vi "Quadratic Roots.vi"() -> ()   [LabVIEW 2021]
panel:
  out "Root 2":dbl
  out "Root 1":dbl
  in  "C":dbl
  in  "B":dbl
  in  "A":dbl
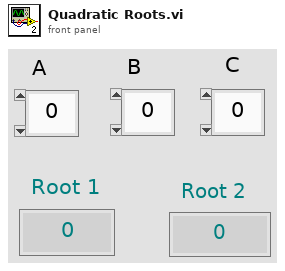
[diagram p1: front panel]
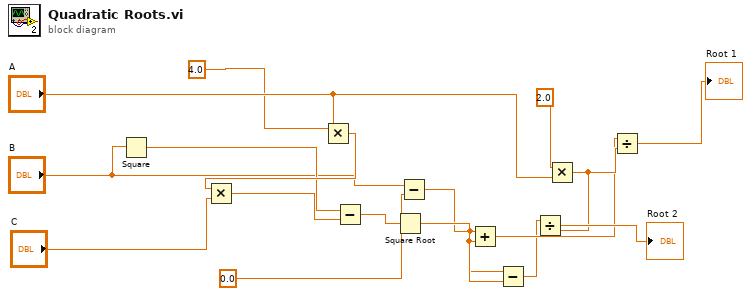
[diagram p0: block diagram]
diagram:
  n1 = Square(x="B") -> (x^2=w15:dbl)
  n2 = Multiply(x=4.0, y="A") -> (x*y=w17:dbl)
  n3 = Multiply(x=w17, y="C") -> (x*y=w14:dbl)
  n4 = Subtract(x=w15, y=w14) -> (x-y=w13:dbl)
  n5 = Square Root(x=w13) -> (sqrt(x)=w7:dbl)
  n6 = Subtract(x="B", y=0.0) -> (x-y=w6:dbl)
  n7 = Add(x=w6, y=w7) -> (x+y=w8:dbl)
  n8 = Subtract(x=w6, y=w7) -> (x-y=w5:dbl)
  n9 = Multiply(x=2.0, y="A") -> (x*y=w9:dbl)
  n10 = Divide(x=w5, y=w9) -> (x/y=→"Root 2":dbl)
  n11 = Divide(x=w8, y=w9) -> (x/y=→"Root 1":dbl)
